vi "contFFLoop.vi"(1 "Numeric":u8) -> ()   [LabVIEW 2015]
uses:
  lv64_eventdriven2015/board.vis/ESLSCDLL.dll
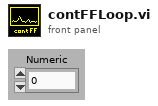
[diagram p1: front panel]
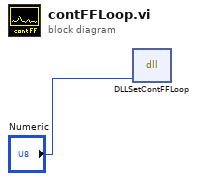
[diagram p0: block diagram]
diagram:
  n1 = dll-call lib="C:/ENTW/PCIE/64bit/lv64/lv64_eventdriven2015/board.vis/ESLSCDLL.dll" fn="DLLSetContFFLoop"("activate"="Numeric") -> ()  [unwired: 5 in, 2 out]
